vi "niRFUtil FTW Generate RBW Response.vi"(0 "Type":T1=enum."Gaussian", 5 "Center Frequency (Hz)":dbl format="%^.2e", 7 "Bandwidth (Hz)":T4 format="%^.3e", 9 "df (Hz)":dbl format="%^.2e", 11 "Minimum Selectivity (dB)":dbl=70.0 format="%.2f") -> (4 "Filter Power Response":T2 {"y" min=0 max=127 format="%.2f"; "dx" format="%^.2e"; "x0" format="%^.2e"}, 6 "-ENBW (dB-Hz)":sgl format="%.2f")   [LabVIEW 2015, in "niRFUtil.lvlib"]
doc: "(c) Copyright 2006, National Instruments, Inc. This VI may not be duplicated, sold, or distributed without written consent from National Instruments."
uses:
  niRFUtil.lvlib
  Includes/niRFUtil INC RBW Filter Bandwidth.ctl
  Includes/niRFUtil INC Real Waveform.ctl
  Includes/niRFUtil INC Real Array.ctl
  Includes/niRFUtil INC RBW Filter Type (Freq Domain).ctl
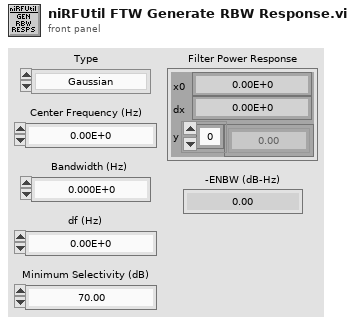
[diagram p1: front panel]
types:
  T1 = typedef "niRFUtil.lvlib/niRFUtil INC RBW Filter Type (Freq Domain).ctl" = enum16{"FFT Based", "Gaussian", "Flat", "Synch Tuned - 4", "Synch Tuned - 5"}
  T2 = typedef "niRFUtil.lvlib/niRFUtil INC Real Waveform.ctl" = cluster{"x0":dbl, "dx":dbl, "y":T3}
  T3 = typedef "niRFUtil.lvlib/niRFUtil INC Real Array.ctl" = sgl[]
  T4 = typedef "niRFUtil.lvlib/niRFUtil INC RBW Filter Bandwidth.ctl" = dbl
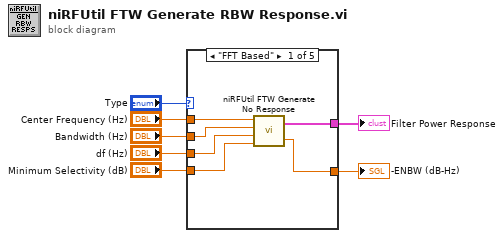
[diagram p0: block diagram]
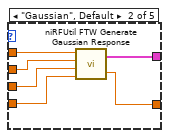
[diagram p2: hidden frame]
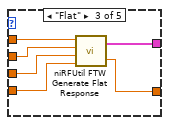
[diagram p3: hidden frame]
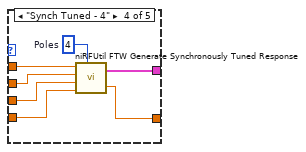
[diagram p4: hidden frame]
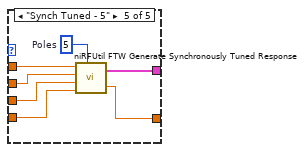
[diagram p5: hidden frame]
diagram:
  n1 = case shown="\"FFT Based\"" "Type" {
    tunnel: "Center Frequency (Hz)" -> [w13 w19 w25 w32 w39]
    tunnel: "Bandwidth (Hz)" -> [w12 w18 w24 w31 w38]
    tunnel: "df (Hz)" -> [w11 w17 w23 w30 w37]
    tunnel: "Minimum Selectivity (dB)" -> [w10 w16 w22 w29 w36]
    tunnel: [w9 w15 w21 w28 w35] -> w2
    tunnel: [w8 w14 w20 w27 w34] -> w1
    frame "FFT Based" {
      n2 = call "niRFUtil FTW Generate No Response.vi"("Minimum Selectivity (dB)"=w10, "df (Hz)"=w11, "Bandwidth (Hz)"=w12, "Center Frequency (Hz)"=w13) -> ("-ENBW (dB-Hz)"=w8:sgl, "Filter Power Response"=w9:T2)
    }
    frame "Gaussian", Default {
      n3 = call "niRFUtil FTW Generate Gaussian Response.vi"("Minimum Selectivity (dB)"=w16, "df (Hz)"=w17, "Bandwidth (Hz)"=w18, "Center Frequency (Hz)"=w19) -> ("-ENBW (dB-Hz)"=w14:sgl, "Filter Power Response"=w15:T2)
    }
    frame "Flat" {
      n4 = call "niRFUtil FTW Generate Flat Response.vi"("Minimum Selectivity (dB)"=w22, "df (Hz)"=w23, "Bandwidth (Hz)"=w24, "Center Frequency (Hz)"=w25) -> ("-ENBW (dB-Hz)"=w20:sgl, "Filter Power Response"=w21:T2)
    }
    frame "Synch Tuned - 4" {
      w26 = 4  # Poles
      n5 = call "niRFUtil FTW Generate Synchronously Tuned Response.vi"("Center Frequency (Hz)"=w32, "Bandwidth (Hz)"=w31, "df (Hz)"=w30, "Minimum Selectivity (dB)"=w29, "Poles (5)"=w26) -> ("Filter Power Response"=w28:T2, "-ENBW (dB-Hz)"=w27:sgl)
    }
    frame "Synch Tuned - 5" {
      w33 = 5  # Poles
      n6 = call "niRFUtil FTW Generate Synchronously Tuned Response.vi"("Center Frequency (Hz)"=w39, "Bandwidth (Hz)"=w38, "df (Hz)"=w37, "Minimum Selectivity (dB)"=w36, "Poles (5)"=w33) -> ("Filter Power Response"=w35:T2, "-ENBW (dB-Hz)"=w34:sgl)
    }
  }
  "Filter Power Response" <- w2
  "-ENBW (dB-Hz)" <- w1
